vi "calculate_drivable_paths_line (test).vi"(11 "allowed proximity squared":i16=100) -> ()   [LabVIEW 2010]
uses:
  <vilib>/rvi/DataTransferAndStorage/Container/XNode/niFpgaContainer.xnode
  athena FPGA globals.vi
  Deleteme/line driveable paths global.vi
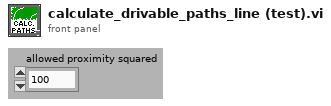
[diagram p1: front panel]
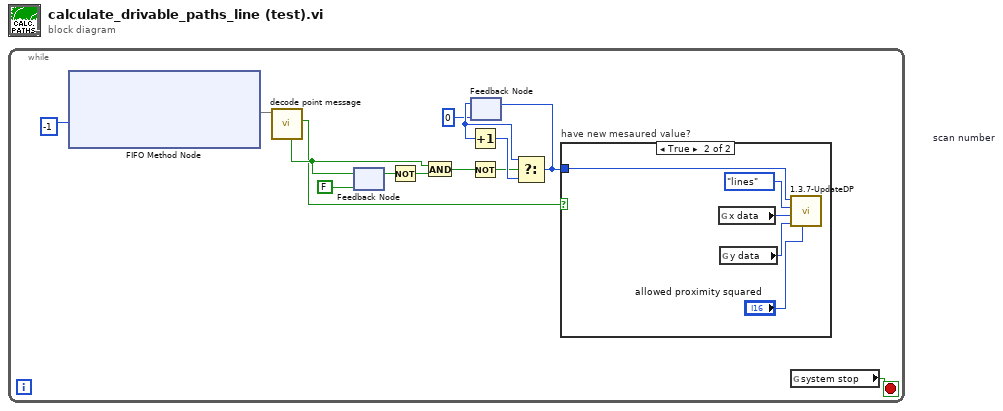
[diagram p0: block diagram]
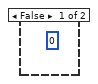
[diagram p2: hidden frame]
diagram:
  n1 = while {
    stop <- w13 stop-if-true
    n2 = xnode ("FIFO Method Node")("Timeout"=-1) -> ("Element"=w4)  [unwired: 1 in, 2 out]
    n3 = call "decode point message.vi"("input stream"=w4) -> ("new y"=w1:bool, "waiting for new message"=w2:bool)  [unwired: 7 in, 2 out]
    n4 = feedback-in #1(w2) -> ()
    n5 = feedback #1(FALSE) -> (w3:bool)
    n6 = Not(x=w3) -> (.not. x?=w12:bool)
    n7 = And(x=w2, y=w12) -> (x .and. y?=w11:bool)
    n8 = Not(x=w11) -> (.not. x?=w6:bool)
    n9 = feedback #2 "scan number"(u8 0 ("y")) -> (w9:u8)
    n10 = Increment(x=w9) -> (x+1=w8:u8)
    n11 = Select(t=w9, s=w6, f=w8) -> (s? t:f=w5:u8)
    n12 = feedback-in #2(w5) -> ()
    n13 = case "have new mesaured value?" shown="True" w1 {
      tunnel: w5 -> [_ w19]
      frame False {
        (unwired) u8 0 ("y")
      }
      frame True {
        n14 = global read "line driveable paths global.vi" "x data"() -> (w15:i16)
        n15 = global read "line driveable paths global.vi" "y data"() -> (w16:i16)
        n16 = call "1.3.7-UpdateDP.vi"("allowed proximity squared"="allowed proximity squared", "Robot Y"=w16, "Robot X"=w15, "update lines or objects"=enum16{"lines", "obstacles"}."lines", "Scan Number"=w19) -> ()  [unwired: 7 in]
      }
    }
    n17 = global read "athena FPGA globals.vi" "system stop"() -> (w13:bool)
  }
